vi "Write Current Paths.vi"(10 "Current Paths":T1(array[cluster]), 11 "PathControl in":refnum<class "PathControl.lvclass">) -> (3 "PathControl out":refnum<class "PathControl.lvclass">)   [LabVIEW 2020, in "PathControl.lvclass"]
uses:
  PathControl.lvclass
  PathControl.lvclass/PathControl.ctl
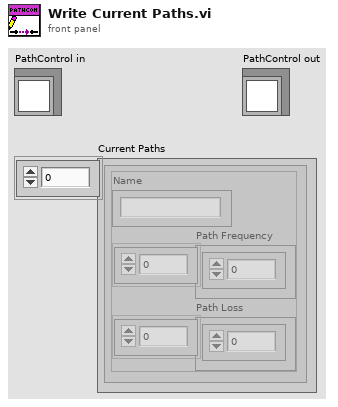
[diagram p1: front panel]
types:
  T1 = cluster{"Name":string, "Path Frequency":dbl[], "Path Loss":dbl[]}[]
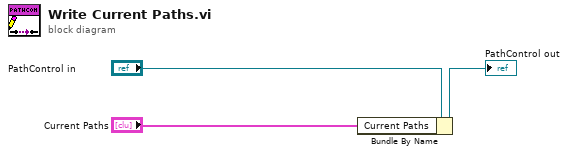
[diagram p0: block diagram]
diagram:
  n1 = Bundle By Name(cluster="PathControl in", "Current Paths"="Current Paths") -> (→"PathControl out":refnum<class "PathControl.lvclass">)
